vi "Current VI Reference.vi"   [LabVIEW 2017]
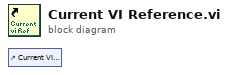
[diagram p0: block diagram]
diagram:
  n1 = control-ref of="Current VI Reference"() -> ()  [unwired: 1 out]
